vi "Write Button Lists Properties.vi"(8 "error in (no error)":errorcluster, 10 "Button Lists Properties":T1[](array[typedef]), 11 "CustomDeviceRepo in":refnum<class "CustomDeviceRepo.lvclass">) -> (0 "error out":errorcluster, 3 "CustomDeviceRepo out":refnum<class "CustomDeviceRepo.lvclass">)   [LabVIEW 2014, in "CustomDeviceRepo.lvclass"]
uses:
  CustomDeviceRepo.lvclass
  Custom Device Type Defs/ButtonLists Properties.ctl
  Custom Device XML/Custom Device XML/Path Cluster.ctl
  Custom Device XML/Custom Device XML/Button Type.ctl
  Custom Device XML/Custom Device XML/Dependency three item small.ctl
  CustomDeviceRepo.lvclass/CustomDeviceRepo.ctl
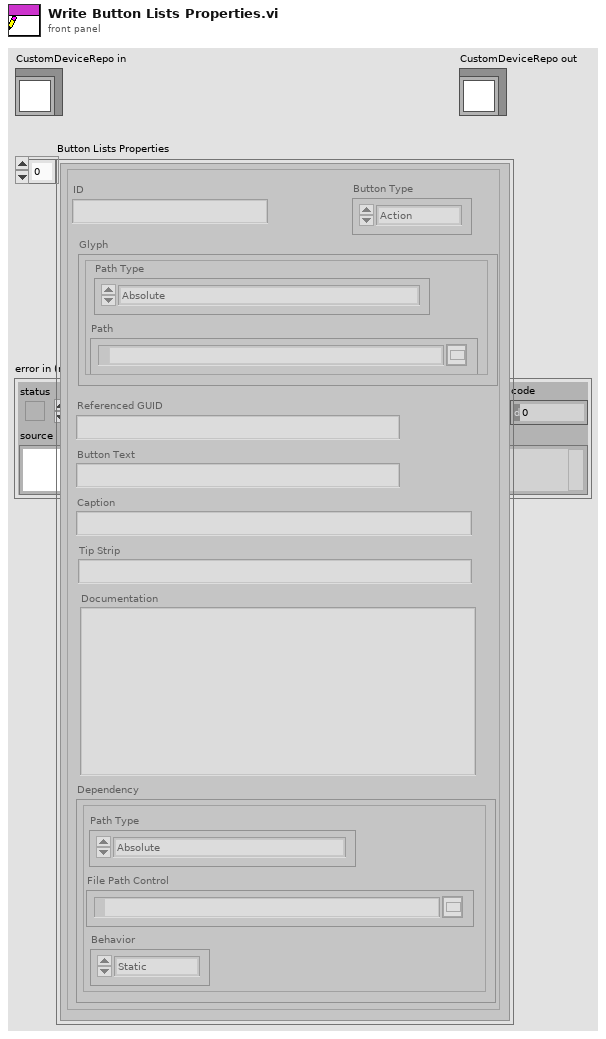
[diagram p1: front panel]
types:
  T1 = typedef "ButtonLists Properties.ctl" = cluster{"ID":string, "Glyph":T2, "Button Type":T3, "Referenced GUID":string, "Button Text":string, "Caption":string, "Tip Strip":string, "Documentation":string, "Dependency":T4}
  T2 = typedef "Path Cluster.ctl" = cluster{"Path":path, "Path Type":enum16{"Absolute", "To Base", "To Common Doc Dir", "To Application Data Dir"}}
  T3 = typedef "Button Type.ctl" = enum16{"Action", "Dialog", "Page", "Notification", "Separator"}
  T4 = typedef "Dependency three item small.ctl" = cluster{"File Path Control":path, "Path Type":enum16{"Absolute", "To Base", "To Common Doc Dir", "To Application Data Dir"}, "Behavior":enum16{"Static", "Dynamic"}}
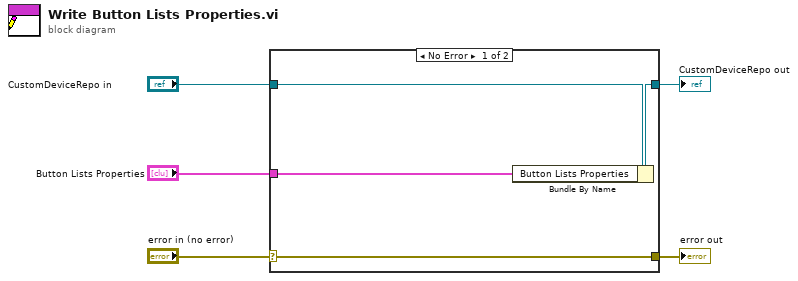
[diagram p0: block diagram]
diagram:
  n1 = case shown="No Error" "error in (no error)" {
    selector: "error in (no error)" -> [w9 w10]
    tunnel: [w9 w10] -> w4
    tunnel: [w7 w11] -> w2
    tunnel: "CustomDeviceRepo in" -> [w8 w11]
    tunnel: "Button Lists Properties" -> [w6 _]
    frame No Error {
      n2 = Bundle By Name(cluster=w8, "Button Lists Properties"=w6) -> (w7:refnum<class "CustomDeviceRepo.lvclass">)
    }
    frame Error {
    }
  }
  "error out" <- w4
  "CustomDeviceRepo out" <- w2
